vi "电压-位移.vi"(11 "输出电压":dbl) -> (3 "位移":dbl)   [LabVIEW 2018]
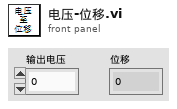
[diagram p1: front panel]
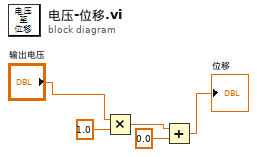
[diagram p0: block diagram]
diagram:
  n1 = Multiply(x="输出电压", y=1.0) -> (x*y=w1:dbl)
  n2 = Add(x=w1, y=0.0) -> (x+y=→"位移":dbl)
